vi "ReadExample.vi"() -> ()   [LabVIEW 2017]
uses:
  <vilib>/UPVI/lvhdf5/dataspace.llb/H5S_seloper_t.ctl
  <vilib>/UPVI/lvhdf5/file.llb/LVH5F Operation.ctl
  <vilib>/UPVI/lvhdf5/dataset.llb/H5Dread (Variant).vi
  <vilib>/UPVI/lvhdf5/library.llb/HDF5 Ref.ctl
  <vilib>/UPVI/lvhdf5/dataset.llb/H5Dread.xnode
  <vilib>/UPVI/lvhdf5/dataset.llb/Simple H5Dread.xnode
  <vilib>/UPVI/lvhdf5/attribute.llb/Simple H5Aread.xnode
  <vilib>/UPVI/lvhdf5/attribute.llb/Simple H5Aread (Variant).vi
  <vilib>/UPVI/lvhdf5/dataspace.llb/LVH5Screate_matching_space.xnode
  <vilib>/UPVI/lvhdf5/dataspace.llb/H5S_class_t.ctl
  <vilib>/UPVI/lvhdf5/dataspace.llb/H5Screate.vi
  <vilib>/UPVI/lvhdf5/dataspace.llb/H5Screate_simple.vi
  <vilib>/UPVI/lvhdf5/dataspace.llb/LVH5Screate_matching_space (Variant).vi
  <vilib>/Utility/miscctls.llb/LVRectTypeDef.ctl
  <vilib>/UPVI/lvhdf5/file.llb/H5Fopen.vi
  <vilib>/UPVI/lvhdf5/group.llb/H5G_obj_t.ctl
  <vilib>/UPVI/lvhdf5/dataset.llb/LVH5D Operation.ctl
  <vilib>/UPVI/lvhdf5/utility.llb/Select HDF5 Dialog.vi
  <vilib>/UPVI/lvhdf5/utility.llb/Select HDF5 Dialog (File and Object).vi
  <vilib>/UPVI/lvhdf5/utility.llb/Select HDF5 Dialog (Object Only).vi
  <vilib>/UPVI/lvhdf5/identifier.llb/Not an HDF5 Refnum Constant.vi
  <vilib>/UPVI/lvhdf5/dataset.llb/Simple H5Dread (Variant).vi
  <vilib>/UPVI/lvhdf5/dataset.llb/OpenCreateReplace Dataset.vi
  <vilib>/UPVI/lvhdf5/dataspace.llb/H5Sget_simple_extent_dims.vi
  <vilib>/UPVI/lvhdf5/attribute.llb/private/LVH5AreadWDTAttrs.vi
  <vilib>/Utility/error.llb/Error Cluster From Error Code.vi
panel:
  out "Data out":dbl[][][](array[numeric])
  in  "Count":u64[](array[numeric])
  in  "Start":u64[](array[numeric])
  in  "Block":u64[](array[numeric])
  in  "Stride":u64[](array[numeric])
  in  "Operator":T1=1 items=["H5S_SELECT_NOOP"=-1, "H5S_SELECT_SET"=0, "H5S_SELECT_OR"=1, "H5S_SELECT_AND"=2, "H5S_SELECT_XOR"=3, "H5S_SELECT_NOTB"=4, "H5S_SELECT_NOTA"=5, "H5S_SELECT_APPEND"=6, "H5S_SELECT_PREPEND"=7]
  in  "Pointlist":u64[][](array[numeric])
  out "Count 4":i64
  out "Count 3":i64
  out "Count 2":i64
  in  "path 2":path
  out "error out 2":errorcluster
  out "Value":string
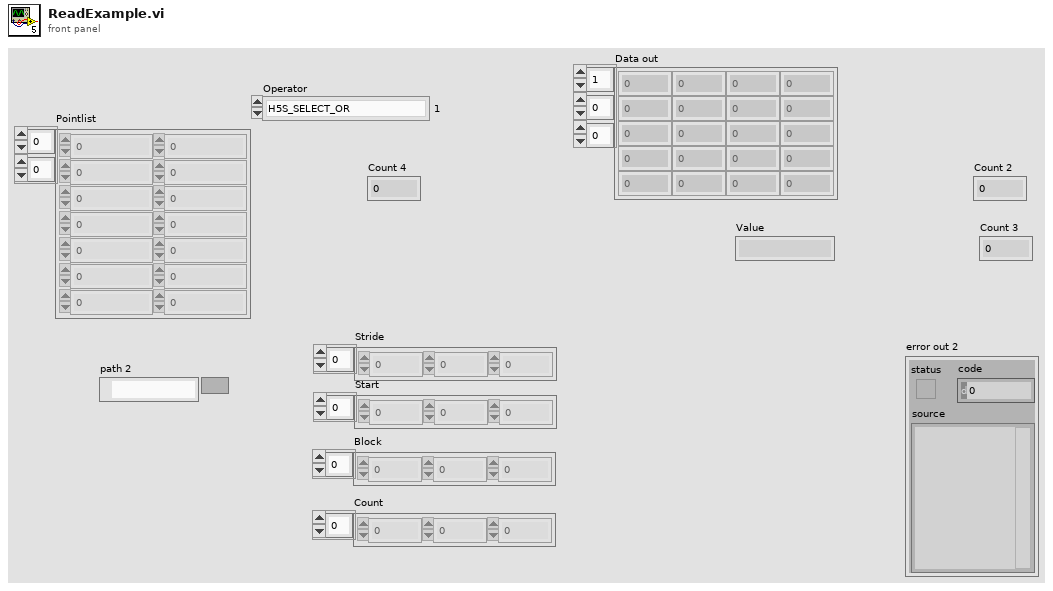
[diagram p1: front panel]
types:
  T1 = typedef "H5S_seloper_t.ctl" = i32
  T2 = typedef "LVH5F Operation.ctl" = enum16{"open", "open or create", "create or replace", "create or replace (with confirmation)", "create", "open (read only)"}
  T3 = typedef "LVRectTypeDef.ctl" = cluster{"Left":i16, "Top":i16, "Right":i16, "Bottom":i16}
  T4 = cluster{"Behavior":enum32{"Invalid", "Default", "Floating", "Floating/Auto-Hide", "Modal"}, "Position":T3, "Center":bool, "Title":string}
  T5 = typedef "LVH5D Operation.ctl" = enum16{"open", "replace", "create", "open or create", "create or replace", "create or replace with confirmation"}
  T6 = typedef "H5G_obj_t.ctl" = i32
  T7 = cluster{"Object Types (any)":T6[], "Object Pattern":string}
  T8 = typedef "HDF5 Ref.ctl" = refnum<k1>
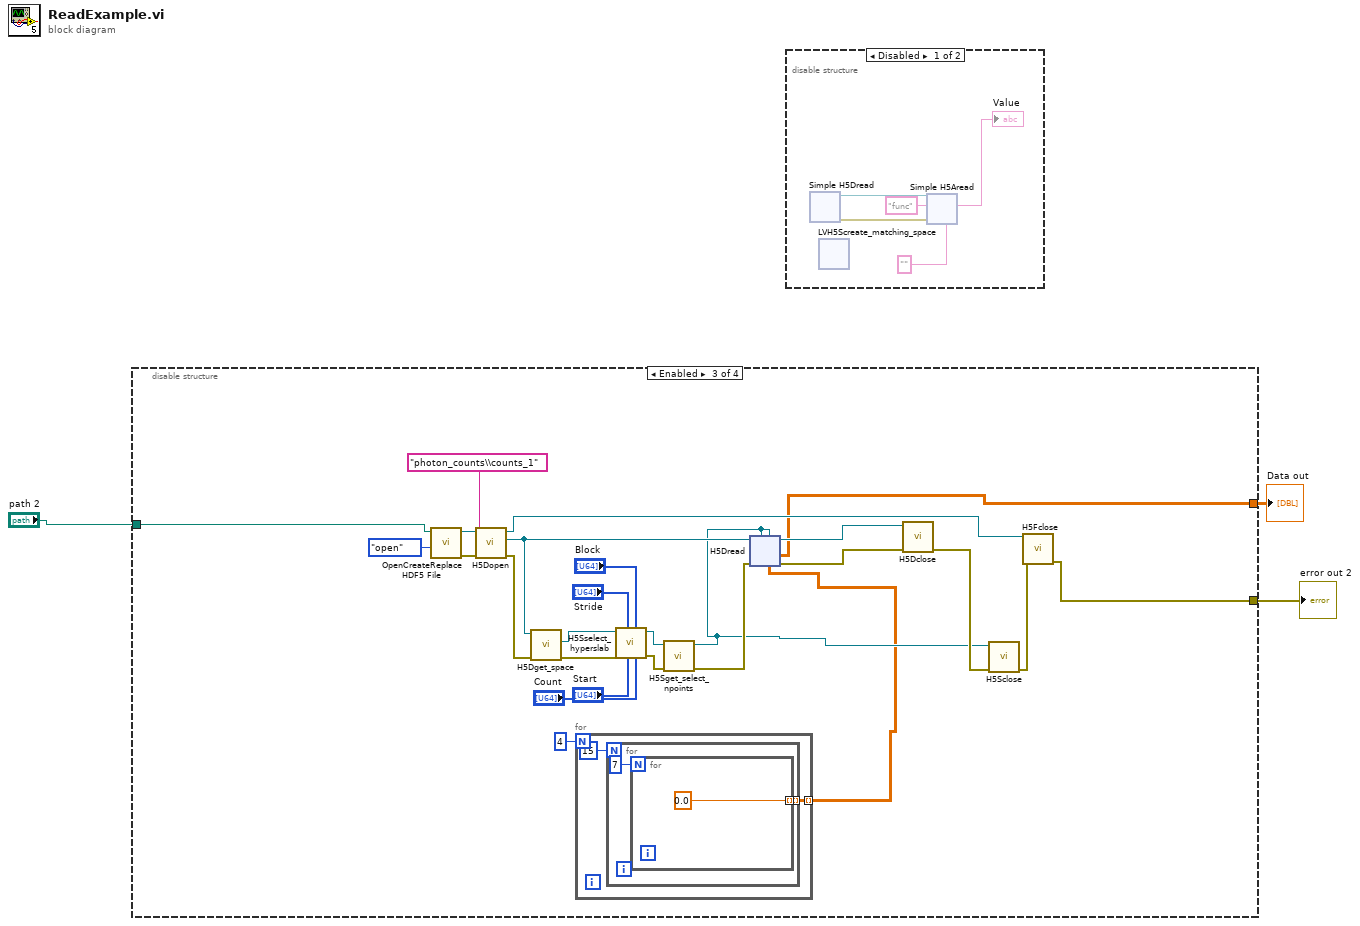
[diagram p0: block diagram]
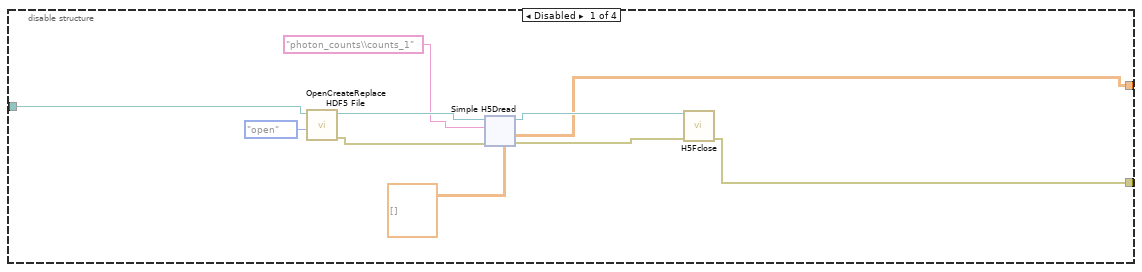
[diagram p2: hidden frame]
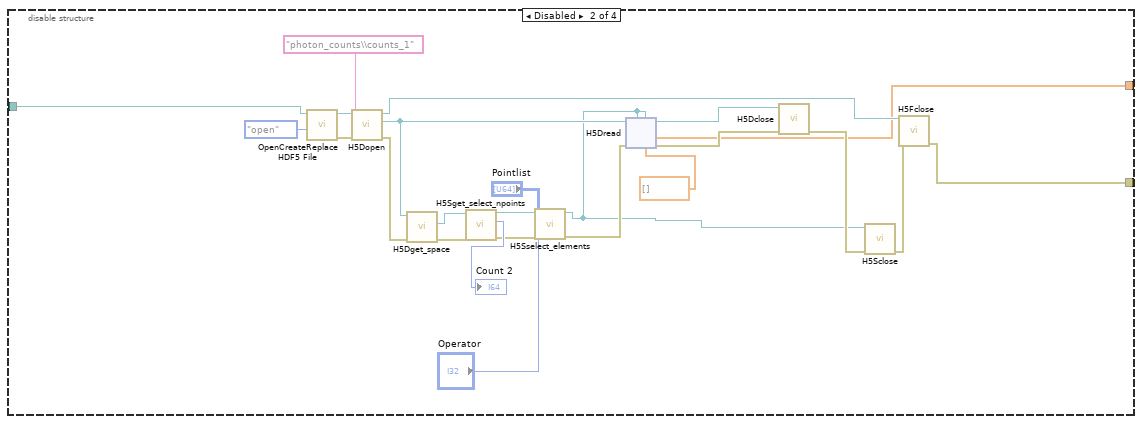
[diagram p3: hidden frame]
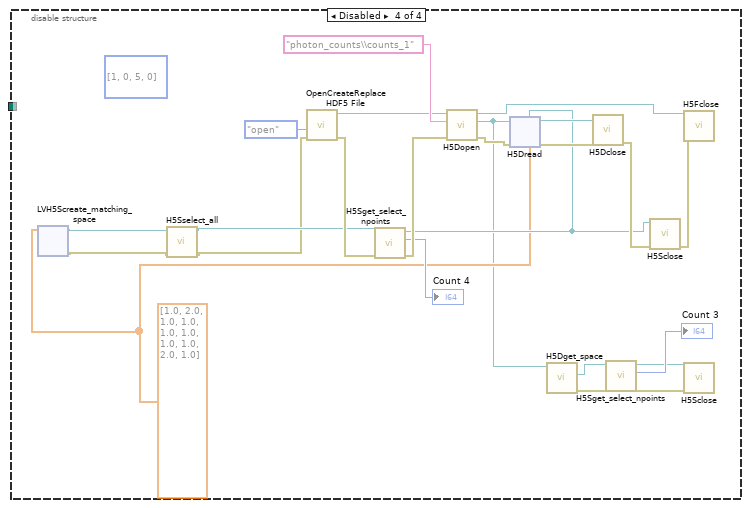
[diagram p4: hidden frame]
diagram:
  n1 = disable-structure shown="Enabled" {
    disable-tunnel: "path 2" -> [w6 w338 w387 _]
    disable-tunnel: [w5 w337 w386 _] -> w1
    disable-tunnel: [w4 w336 w385 _] -> w2
    frame Disabled {
      n2 = call <vilib>:"OpenCreateReplace HDF5 File.vi"("function (open or create)"=LVH5F_Operation."open", "path"=w6) -> ("error out"=w12:errorcluster, "HDF5 Ref out"=w11:T8)  [unwired: 6 in]
      n3 = xnode "Simple H5Dread"("Dataset Path"="photon_counts\\counts_1", "error in (no error)"=w12, "HDF5 Path or Ref"=w11, "Data"=dbl[][][] [] ("Data out 2")) -> ("HDF5 Ref out"=w9:T8, "error out"=w8:errorcluster, "Data out"=w5:dbl[][][])  [unwired: 1 out]
      n4 = call <vilib>:"H5Fclose.vi"("error in (no error)"=w8, "HDF5 Ref"=w9) -> ("error out"=w4:errorcluster)  [unwired: 7 in]
    }
    frame Disabled {
      n5 = call <vilib>:"OpenCreateReplace HDF5 File.vi"("function (open or create)"=LVH5F_Operation."open", "path"=w338) -> ("error out"=w344:errorcluster, "HDF5 Ref out"=w351:T8)  [unwired: 6 in]
      n6 = call <vilib>:"H5Dopen.vi"("error in (no error)"=w344, "name"="photon_counts\\counts_1" ("Dataset Path"), "HDF5 Ref"=w351) -> ("error out"=w341:errorcluster, "HDF5 Dataset Ref"=w342:T8, "HDF5 Ref out"=w339:T8)  [unwired: 4 in]
      n7 = call <vilib>:"H5Dget_space.vi"("error in (no error)"=w341, "HDF5 Dataset Ref"=w342) -> ("error out"=w346:errorcluster, "HDF5 Dataspace Ref"=w343:T8)  [unwired: 5 in, 1 out]
      n8 = call <vilib>:"H5Sget_select_npoints.vi"("error in (no error)"=w346, "HDF5 Space Ref"=w343) -> ("error out"=w334:errorcluster, "Count"=→"Count 2":i64, "HDF5 Ref out"=w335:T8)  [unwired: 5 in]
      n9 = call <vilib>:"H5Sselect_elements.vi"("error in (no error)"=w334, "Pointlist"="Pointlist", "Operator"="Operator", "HDF5 Space Ref"=w335) -> ("error out"=w333:errorcluster, "HDF5 Ref out"=w330:T8)  [unwired: 4 in]
      n10 = xnode "H5Dread"("HDF5 Dataset Ref"=w342, "HDF5 File Space (H5S_ALL)"=w330, "HDF5 Memory Space"=w330, "error in (no error)"=w333, "Data"=dbl[] []) -> ("HDF5 Dataset Ref out"=w348:T8, "error out"=w347:errorcluster, "Data out"=w337:dbl[])  [unwired: 2 in]
      n11 = call <vilib>:"H5Dclose.vi"("error in (no error)"=w347, "HDF5 Dataset Ref"=w348) -> ("error out"=w350:errorcluster)  [unwired: 7 in]
      n12 = call <vilib>:"H5Sclose.vi"("error in (no error)"=w350, "HDF5 Dataspace Ref"=w330) -> ("error out"=w349:errorcluster)  [unwired: 7 in]
      n13 = call <vilib>:"H5Fclose.vi"("error in (no error)"=w349, "HDF5 Ref"=w339) -> ("error out"=w336:errorcluster)  [unwired: 7 in]
    }
    frame Enabled {
      n14 = call <vilib>:"OpenCreateReplace HDF5 File.vi"("function (open or create)"=LVH5F_Operation."open", "path"=w387) -> ("error out"=w391:errorcluster, "HDF5 Ref out"=w396:T8)  [unwired: 6 in]
      n15 = call <vilib>:"H5Dopen.vi"("error in (no error)"=w391, "name"="photon_counts\\counts_1" ("Dataset Path"), "HDF5 Ref"=w396) -> ("error out"=w389:errorcluster, "HDF5 Dataset Ref"=w390:T8, "HDF5 Ref out"=w388:T8)  [unwired: 4 in]
      n16 = call <vilib>:"H5Dget_space.vi"("error in (no error)"=w389, "HDF5 Dataset Ref"=w390) -> ("error out"=w384:errorcluster, "HDF5 Dataspace Ref"=w383:T8)  [unwired: 5 in, 1 out]
      n17 = for {
        N: 4 -> [_]
        tunnel: [w400] -> w373 mode=indexing
        n18 = for {
          N: 15 -> [_]
          tunnel: [w402] -> w400 mode=indexing
          n19 = for {
            N: 7 -> [_]
            tunnel: [0.0] -> w402 mode=indexing
          }
        }
      }
      n20 = call <vilib>:"H5Sselect_hyperslab.vi"("Count"="Count", "Block"="Block", "Start"="Start", "Stride"="Stride", "error in (no error)"=w384, "HDF5 Space Ref"=w383) -> ("error out"=w377:errorcluster, "HDF5 Ref out"=w378:T8)  [unwired: 4 in]
      n21 = call <vilib>:"H5Sget_select_npoints.vi"("error in (no error)"=w377, "HDF5 Space Ref"=w378) -> ("error out"=w376:errorcluster, "HDF5 Ref out"=w374:T8)  [unwired: 5 in, 1 out]
      n22 = xnode "H5Dread"("HDF5 Dataset Ref"=w390, "HDF5 File Space (H5S_ALL)"=w374, "HDF5 Memory Space"=w374, "error in (no error)"=w376, "Data"=w373) -> ("HDF5 Dataset Ref out"=w393:T8, "error out"=w392:errorcluster, "Data out"=w386:dbl[][][])  [unwired: 2 in]
      n23 = call <vilib>:"H5Dclose.vi"("error in (no error)"=w392, "HDF5 Dataset Ref"=w393) -> ("error out"=w395:errorcluster)  [unwired: 7 in]
      n24 = call <vilib>:"H5Sclose.vi"("error in (no error)"=w395, "HDF5 Dataspace Ref"=w374) -> ("error out"=w394:errorcluster)  [unwired: 7 in]
      n25 = call <vilib>:"H5Fclose.vi"("error in (no error)"=w394, "HDF5 Ref"=w388) -> ("error out"=w385:errorcluster)  [unwired: 7 in]
    }
    frame Disabled {
      (unwired) u64[][] [[1, 0], [5, 0]] ("Pointlist")
      w433 = dbl[] [1.0, 2.0, 1.0, 1.0, 1.0, 1.0, 1.0, 1.0, 2.0, 1.0]
      n26 = xnode "LVH5Screate_matching_space"("Data"=w433) -> ("HDF5 Dataspace Ref"=w432:T8, "error out"=w429:errorcluster)  [unwired: 2 in]
      n27 = call <vilib>:"H5Sselect_all.vi"("error in (no error)"=w429, "HDF5 Space Ref"=w432) -> ("error out"=w430:errorcluster, "HDF5 Ref out"=w431:T8)  [unwired: 6 in]
      n28 = call <vilib>:"OpenCreateReplace HDF5 File.vi"("error in (no error)"=w430, "function (open or create)"=LVH5F_Operation."open") -> ("error out"=w446:errorcluster, "HDF5 Ref out"=w444:T8, "path"=w448:path)  [unwired: 5 in]
      n29 = call <vilib>:"H5Sget_select_npoints.vi"("error in (no error)"=w446, "HDF5 Space Ref"=w431) -> ("error out"=w443:errorcluster, "Count"=→"Count 4":i64, "HDF5 Ref out"=w434:T8)  [unwired: 5 in]
      n30 = call <vilib>:"H5Dopen.vi"("error in (no error)"=w443, "name"="photon_counts\\counts_1" ("Dataset Path"), "HDF5 Ref"=w444) -> ("error out"=w435:errorcluster, "HDF5 Dataset Ref"=w428:T8, "HDF5 Ref out"=w442:T8)  [unwired: 4 in]
      n31 = xnode "H5Dread"("HDF5 Dataset Ref"=w428, "HDF5 File Space (H5S_ALL)"=w434, "error in (no error)"=w435, "Data"=w433) -> ("HDF5 Dataset Ref out"=w438:T8, "error out"=w436:errorcluster, "Data out"=w437:dbl[])  [unwired: 3 in]
      n32 = call <vilib>:"H5Dget_space.vi"("HDF5 Dataset Ref"=w428) -> ("error out"=w427:errorcluster, "HDF5 Dataspace Ref"=w423:T8)  [unwired: 6 in, 1 out]
      n33 = call <vilib>:"H5Dclose.vi"("error in (no error)"=w436, "HDF5 Dataset Ref"=w438) -> ("error out"=w441:errorcluster)  [unwired: 7 in]
      n34 = call <vilib>:"H5Sget_select_npoints.vi"("error in (no error)"=w427, "HDF5 Space Ref"=w423) -> ("error out"=w424:errorcluster, "Count"=→"Count 3":i64, "HDF5 Ref out"=w425:T8)  [unwired: 5 in]
      n35 = call <vilib>:"H5Sclose.vi"("error in (no error)"=w441, "HDF5 Dataspace Ref"=w434) -> ("error out"=w440:errorcluster)  [unwired: 7 in]
      n36 = call <vilib>:"H5Fclose.vi"("error in (no error)"=w440, "HDF5 Ref"=w442) -> ()  [unwired: 7 in, 1 out]
      n37 = call <vilib>:"H5Sclose.vi"("error in (no error)"=w424, "HDF5 Dataspace Ref"=w425) -> ()  [unwired: 7 in, 1 out]
    }
  }
  "error out 2" <- w2
  "Data out" <- w1
  n38 = disable-structure shown="Disabled" {
    frame Disabled {
      n39 = xnode "Simple H5Dread"() -> ("HDF5 Ref out"=w517:T8, "error out"=w516:errorcluster)  [unwired: 4 in, 2 out]
      n40 = xnode "LVH5Screate_matching_space"() -> ()  [unwired: 3 in, 2 out]
      n41 = xnode "Simple H5Aread"("HDF5 Ref"=w517, "Name"="func", "error in (no error)"=w516, "Type"="") -> ("Value"=→"Value":string)  [unwired: 2 out]
    }
    frame Enabled {
    }
  }
